vi "Write 4 Audio Track.vi"(6 "Track Enable":T4, 8 "Error In":errorcluster, 9 "Write Position":i64, 10 "4-Track Audio":T2, 11 "Track (File) References In":T1) -> (0 "Error Out":errorcluster, 3 "Track (File) References Out":T1)   [LabVIEW 2015]
doc: "Use this VI to write audio data to a Track file. This function will always write to both Left and Right channels. You must provide the VI with:\n\nTrack File References: Track Ref + Track Name. \n4-Track Audio: The data you want to write.\nTrack Enable: Define which tracks you want to write too. Setting to True will enable writes to this track. \nChannel Write Positions: Can specify a starting\\offset write position for each track you want to write too."
uses:
  Controls/Track Enable.ctl
  Controls/Track (File) References.ctl
  Controls/4 Track Audio.ctl
  Controls/Audio In.ctl
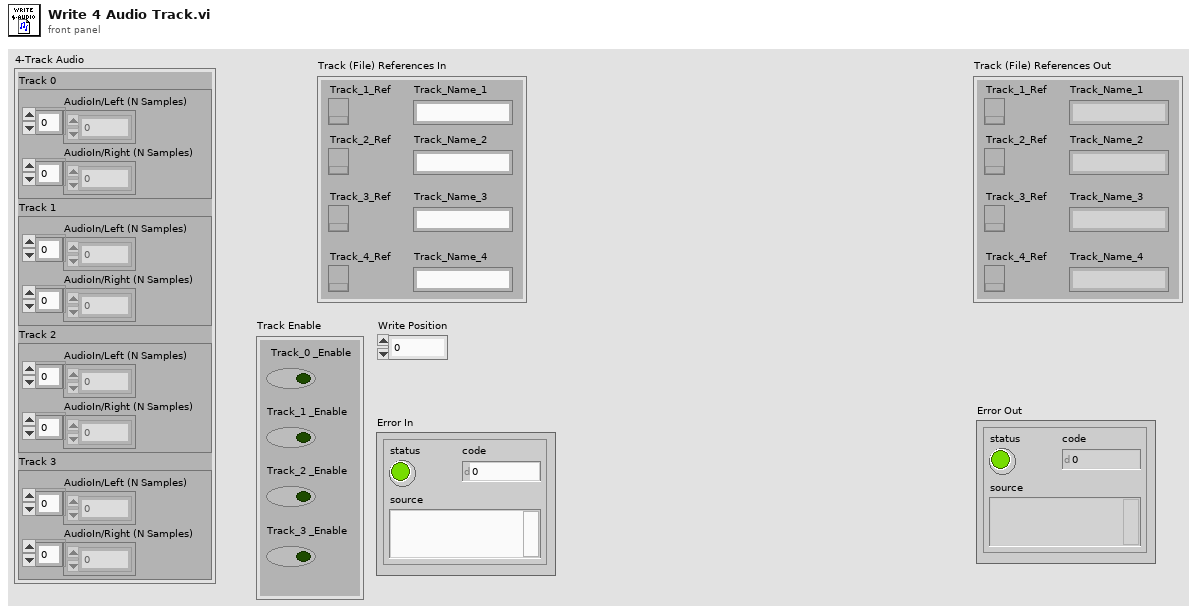
[diagram p1: front panel]
types:
  T1 = typedef "Track (File) References.ctl" = cluster{"Track_1_Ref":refnum<k34>, "Track_2_Ref":refnum<k34>, "Track_3_Ref":refnum<k34>, "Track_4_Ref":refnum<k34>, "Track_Name_1":string, "Track_Name_2":string, "Track_Name_3":string, "Track_Name_4":string}
  T2 = typedef "4 Track Audio.ctl" = cluster{"Track 0":T3, "Track 1":T3, "Track 2":T3, "Track 3":T3}
  T3 = typedef "Audio In.ctl" = cluster{"AudioIn/Left (N Samples)":i16[], "AudioIn/Right (N Samples)":i16[]}
  T4 = typedef "Track Enable.ctl" = cluster{"Track_0 _Enable ":bool, "Track_1 _Enable ":bool, "Track_2 _Enable ":bool, "Track_3 _Enable ":bool}
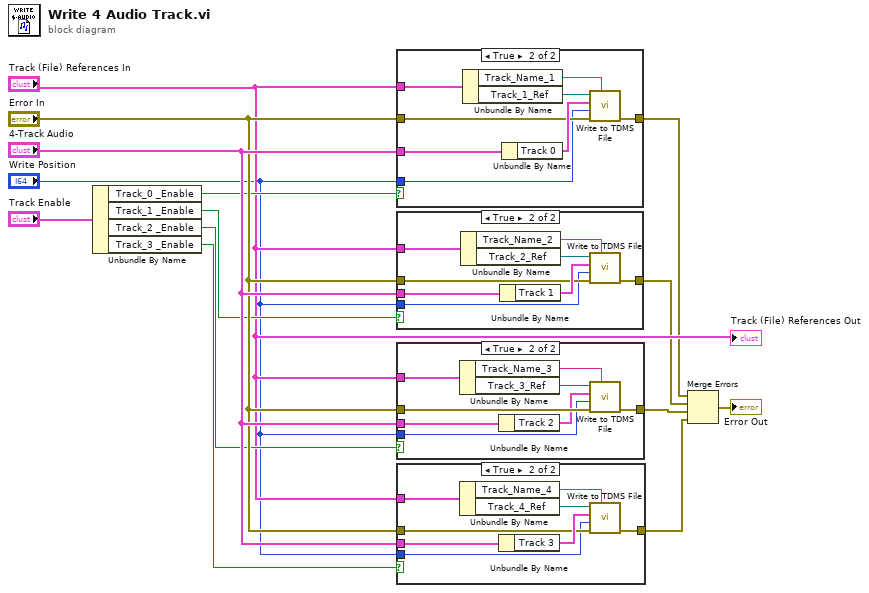
[diagram p0: block diagram]
diagram:
  n1 = Unbundle By Name("Track Enable") -> ("Track_0 _Enable"=w11:bool, "Track_1 _Enable"=w10:bool, "Track_2 _Enable"=w9:bool, "Track_3 _Enable"=w8:bool)
  n2 = case shown="True" w11 {
    tunnel: "4-Track Audio" -> [_ w23]
    tunnel: "Track (File) References In" -> [_ w22]
    tunnel: "Error In" -> [w15 w17]
    tunnel: [w15 w19] -> w6
    tunnel: "Write Position" -> [_ w16]
    frame False {
    }
    frame True {
      n3 = Unbundle By Name(w22) -> ("Track_Name_1"=w21:string, "Track_1_Ref"=w20:refnum<k34>)
      n4 = Unbundle By Name(w23) -> ("Track 0"=w18:T3)
      n5 = call "Write to TDMS File.vi"("Track Name"=w21, "Error In"=w17, "Write Position"=w16, "Audio In"=w18, "TDMS Reference In"=w20) -> ("Error Out"=w19:errorcluster)  [unwired: 5 in, 1 out]
    }
  }
  n6 = case shown="True" w10 {
    tunnel: "4-Track Audio" -> [_ w32]
    tunnel: "Track (File) References In" -> [_ w31]
    tunnel: "Error In" -> [w24 w26]
    tunnel: [w24 w30] -> w5
    tunnel: "Write Position" -> [_ w25]
    frame False {
    }
    frame True {
      n7 = Unbundle By Name(w31) -> ("Track_Name_2"=w29:string, "Track_2_Ref"=w28:refnum<k34>)
      n8 = Unbundle By Name(w32) -> ("Track 1"=w27:T3)
      n9 = call "Write to TDMS File.vi"("Track Name"=w29, "Error In"=w26, "Write Position"=w25, "Audio In"=w27, "TDMS Reference In"=w28) -> ("Error Out"=w30:errorcluster)  [unwired: 5 in, 1 out]
    }
  }
  n10 = case shown="True" w9 {
    tunnel: "4-Track Audio" -> [_ w41]
    tunnel: "Track (File) References In" -> [_ w40]
    tunnel: "Error In" -> [w33 w36]
    tunnel: [w33 w39] -> w4
    tunnel: "Write Position" -> [_ w34]
    frame False {
    }
    frame True {
      n11 = Unbundle By Name(w40) -> ("Track_Name_3"=w38:string, "Track_3_Ref"=w37:refnum<k34>)
      n12 = Unbundle By Name(w41) -> ("Track 2"=w35:T3)
      n13 = call "Write to TDMS File.vi"("Track Name"=w38, "Error In"=w36, "Write Position"=w34, "Audio In"=w35, "TDMS Reference In"=w37) -> ("Error Out"=w39:errorcluster)  [unwired: 5 in, 1 out]
    }
  }
  n14 = case shown="True" w8 {
    tunnel: "4-Track Audio" -> [_ w50]
    tunnel: "Track (File) References In" -> [_ w49]
    tunnel: "Error In" -> [w42 w44]
    tunnel: [w42 w48] -> w3
    tunnel: "Write Position" -> [_ w43]
    frame False {
    }
    frame True {
      n15 = Unbundle By Name(w49) -> ("Track_Name_4"=w47:string, "Track_4_Ref"=w46:refnum<k34>)
      n16 = Unbundle By Name(w50) -> ("Track 3"=w45:T3)
      n17 = call "Write to TDMS File.vi"("Track Name"=w47, "Error In"=w44, "Write Position"=w43, "Audio In"=w45, "TDMS Reference In"=w46) -> ("Error Out"=w48:errorcluster)  [unwired: 5 in, 1 out]
    }
  }
  n18 = Merge Errors(w6, w5, w4, w3) -> (→"Error Out":errorcluster)
  "Track (File) References Out" <- "Track (File) References In"
